vi "Get Name.vi"(11 "Database UI in":refnum<class "Database Provider.lvclass">) -> (2 "Name":string, 3 "Database UI out":refnum<class "Database Provider.lvclass">)   [LabVIEW 2023, in "Database Provider.lvlib" / "Database Provider.lvclass"]
uses:
  Database Provider.lvclass
  Database Provider.lvclass/Database Provider.ctl
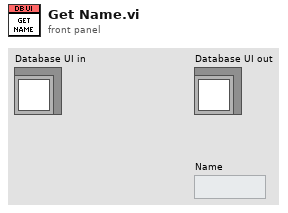
[diagram p1: front panel]
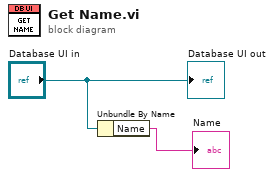
[diagram p0: block diagram]
diagram:
  n1 = Unbundle By Name("Database UI in") -> ("Name"=→"Name":string)
  "Database UI out" <- "Database UI in"
